vi "Unclaimed LVClass Check.vi"(10 "Claimed Class":path[](array[path]), 11 "Class Path List In":path[](array[path])) -> (3 "Class Path List Out":path[](array[path]))   [LabVIEW 2019, in "DepsWatch.lvlib"]
uses:
  DepsWatch.lvlib
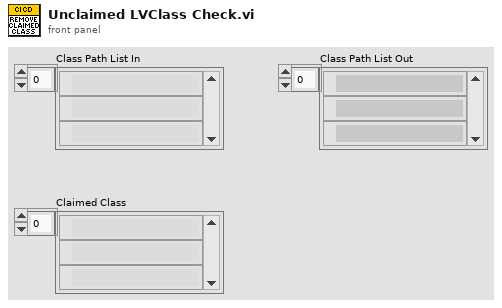
[diagram p1: front panel]
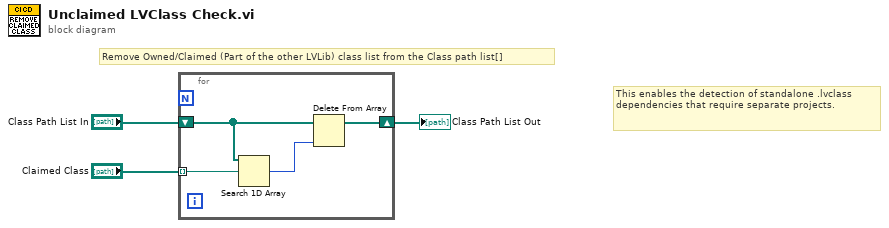
[diagram p0: block diagram]
diagram:
  # "This enables the detection of standalone .lvclass dependencies that require separate projects."
  # "Remove Owned/Claimed (Part of the other LVLib) class list from the Class path list[]"
  n1 = for {
    shift-right: [w4] -> w2
    shift-left: "Class Path List In" -> [w6]
    tunnel: "Claimed Class" -> [w7] mode=indexing
    n2 = Search 1D Array(1D array=w6, element=w7) -> (index of element=w5:i32)  [unwired: 1 in]
    n3 = Delete From Array(array=w6, index=w5) -> (array with subset deleted=w4:path[])  [unwired: 1 in, 1 out]
  }
  "Class Path List Out" <- w2
